vi "写入数据库.vi"(7 "SERVER(IP)":string="PC-WEILY\\SQLEXPRESS", 8 "error in":errorcluster, 9 "values":string, 11 "测试项目":string) -> (0 "error out":errorcluster)   [LabVIEW 2020]
uses:
  LabSQL ADO functions/Ctl/database_Method.ctl
panel:
  in  "Table":string="airtest"
  in  "DATABASE":string="packcode"
  in  "PWD":string="Dmegc@123"
  in  "UID":string="sa"
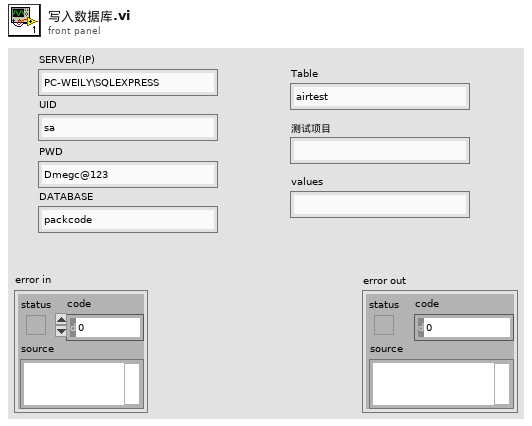
[diagram p1: front panel]
types:
  T1 = typedef "database_Method.ctl" = enum16{"初始化", "查询", "关闭"}
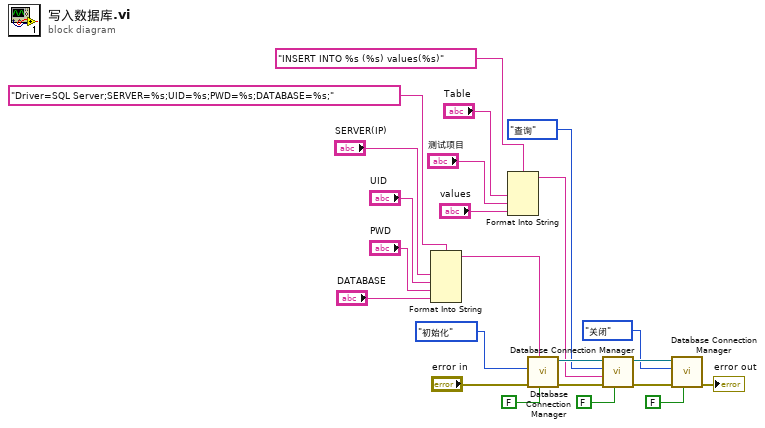
[diagram p0: block diagram]
diagram:
  n1 = Format Into String(format string="Driver=SQL Server;SERVER=%s;UID=%s;PWD=%s;DATABASE=%s;" ("ConnectionString"), "SERVER(IP)", "UID", "PWD", "DATABASE") -> (resulting string=w7:string)  [unwired: 2 in, 1 out]
  n2 = Format Into String(format string="INSERT INTO %s (%s) values(%s)" ("Command Text"), "Table", "测试项目", "values") -> (resulting string=w4:string)  [unwired: 2 in, 1 out]
  n3 = call "Database Connection Manager.vi"("Return Data (T)"=FALSE, "ConnectionString"=w7, "error in (no error)"="error in", "Method"=database_Method."初始化") -> ("error out"=w21:errorcluster, "ADODB._Connection Out"=w20:refnum<k7>)  [unwired: 4 in, 2 out]
  n4 = call "Database Connection Manager.vi"("Return Data (T)"=FALSE, "error in (no error)"=w21, "Command Text"=w4, "Method"=database_Method."查询", "ADODB._Connection In"=w20) -> ("error out"=w17:errorcluster, "ADODB._Connection Out"=w16:refnum<k7>)  [unwired: 3 in, 2 out]
  n5 = call "Database Connection Manager.vi"("Return Data (T)"=FALSE, "error in (no error)"=w17, "Method"=database_Method."关闭", "ADODB._Connection In"=w16) -> ("error out"=→"error out":errorcluster)  [unwired: 4 in, 3 out]
